vi "Calibrate Image.vi"(7 "Calibrate":bool, 8 "error in (no error)":errorcluster, 9 "Internal Parameters":T1, 10 "Camera Name":string="cam0", 11 "Image In":T2) -> (0 "error out":errorcluster, 3 "Image Out":T2)   [LabVIEW 2025]
uses:
  <vilib>/vision/Image Controls.llb/IMAQ Image.ctl
  <vilib>/vision/Calibration.llb/Internal Parameters.ctl
  <vilib>/vision/NI_Vision_Development_Module.lvlib
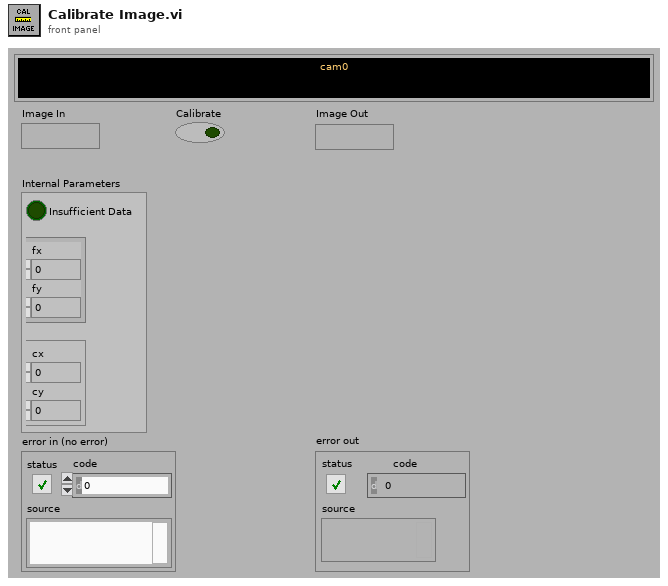
[diagram p1: front panel]
types:
  T1 = typedef "Internal Parameters.ctl" = cluster{"Insufficient Data":bool, "Focal Length (pixel)":cluster{"fx":sgl, "fy":sgl}, "Optical Center (pixel)":cluster{"cx":sgl, "cy":sgl}}
  T2 = typedef "IMAQ Image.ctl" = refnum<image>
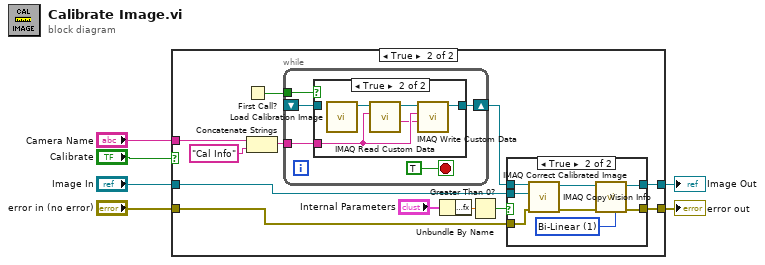
[diagram p0: block diagram]
diagram:
  n1 = case shown="True" "Calibrate" {
    tunnel: [w7 w20] -> w6
    tunnel: "Image In" -> [w7 w19]
    tunnel: "error in (no error)" -> [w8 w18]
    tunnel: [w8 w14] -> w3
    tunnel: "Camera Name" -> [_ w9]
    frame False {
    }
    frame True {
      n2 = First Call?() -> (First Call?: T/F=w13:bool)
      n3 = Concatenate Strings(w9, "Cal Info" ("Image Name")) -> (w11:string)
      n4 = while {
        shift-right: [w25] -> w12
        shift-left: _ -> [w23]
        tunnel: w13 -> [w24]
        tunnel: w11 -> [w21]
        stop <- TRUE stop-if-true
        n5 = case shown="True" w24 {
          tunnel: [w26 w27] -> w25
          tunnel: w23 -> [w26 _]
          tunnel: w21 -> [_ w31]
          frame False {
          }
          frame True {
            n6 = call "Load Calibration Image.vi"() -> ("Image Out"=w28:T2)  [unwired: 7 in, 4 out]
            n7 = call "IMAQ Read Custom Data"("Key"=w31, "Image"=w28) -> ("Custom Data Out"=w29:string, "Image (duplicate)"=w30:T2)  [unwired: 7 in, 1 out]
            n8 = call "IMAQ Write Custom Data"("Custom Data In"=w29, "Key"=w31, "Image"=w30) -> ("Image Out"=w27:T2)  [unwired: 7 in, 1 out]
          }
        }
      }
      n9 = Unbundle By Name("Internal Parameters") -> ("Focal Length (pixel).fx"=w17:sgl)
      n10 = Greater Than 0?(x=w17) -> (x > 0?=w16:bool)
      n11 = case shown="True" w16 {
        tunnel: [w32 w36] -> w14
        tunnel: [w33 w35] -> w20
        tunnel: w19 -> [w33 w40]
        tunnel: w12 -> [_ w41]
        tunnel: w18 -> [w32 w38]
        frame False {
        }
        frame True {
          w34 = u32 1 items=["Zero Order", "Bi-Linear", "Quadratic", "Cubic Spline"] ("Interpolation Type")
          n12 = call "IMAQ Copy Vision Info"("error in (no error)"=w38, "Image Dst"=w40, "Image Src"=w41) -> ("error out"=w37:errorcluster, "Image Dst Out"=w39:T2)  [unwired: 6 in, 1 out]
          n13 = call "IMAQ Correct Calibrated Image"("Interpolation Type"=w34, "error in (no error)"=w37, "Image Src"=w39) -> ("error out"=w36:errorcluster, "Corrected Image"=w35:T2)  [unwired: 7 in]
        }
      }
    }
  }
  "error out" <- w3
  "Image Out" <- w6
